vi "Launcher.vi"() -> ()   [LabVIEW 2025]
doc: "This is the top-level VI of this application. When it runs, it behaves like the splash screen many applications use to keep the user occupied while the application loads into memory. This application is quite small, so there is little overhead, which would make the splash screen just flash for a moment. Because that flash is distracting, there is a three-second delay inserted into this VI so that it stays up for a little bit. \n\nThis VI uses a delay-loaded subVI call to load the rest of the application. This trick ensures that the splash screen can load instantly regardless of how large the rest of the VI hierarchy gets, and the loading of the rest of the VIs becomes one step in the load process."
uses:
  Configuration Tools/Config Tool.lvlib
  Configuration Tools/SubVI/Load App.vi
panel:
  out "Engine Status":i32(listbox)=-1
  out "Title":string
  out "String":string
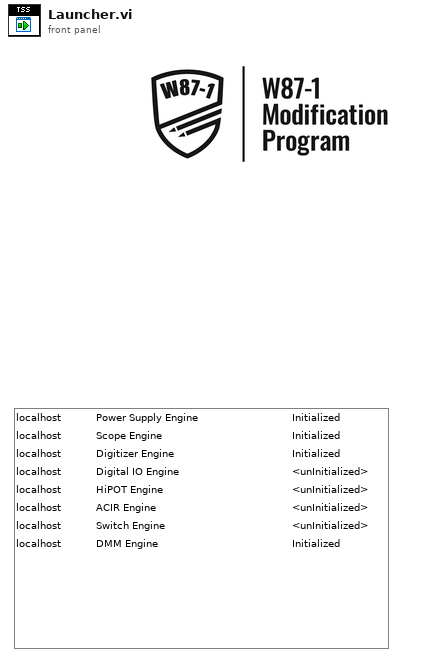
[diagram p1: front panel]
types:
  T1 = enum32{"Invalid", "Default", "Floating", "Floating/Auto-Hide", "Modal"}
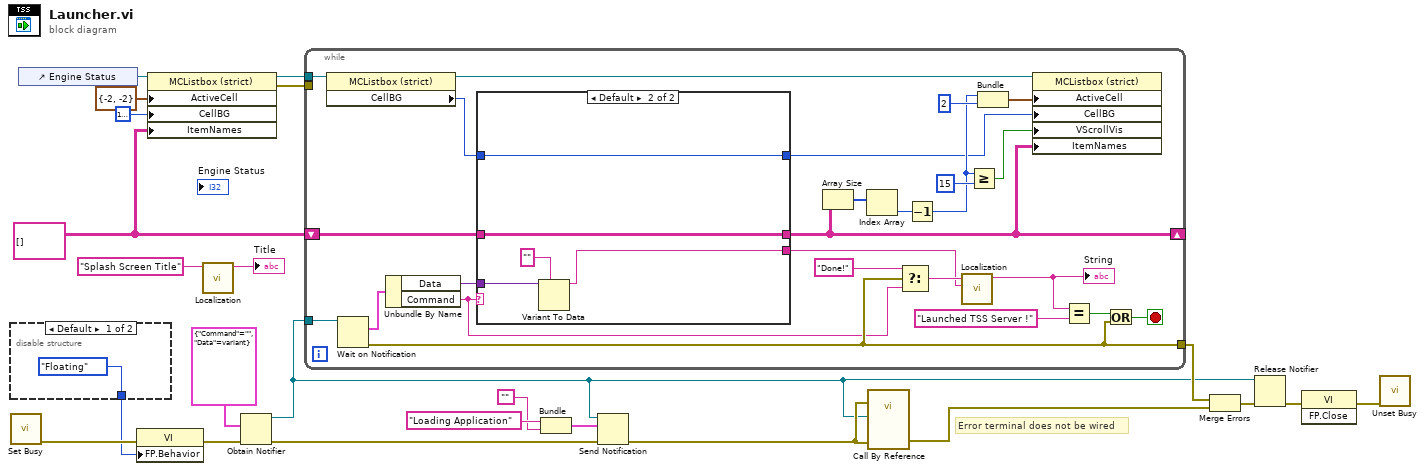
[diagram p0: block diagram]
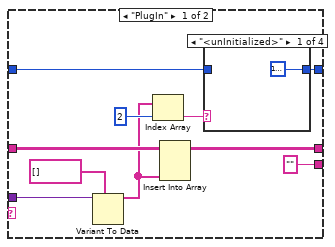
[diagram p2: hidden frame]
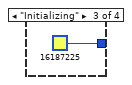
[diagram p4: hidden frame]
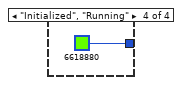
[diagram p5: hidden frame]
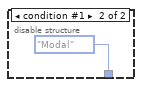
[diagram p6: hidden frame]
diagram:
  w4 = string[][] [] ("ItemNames")
  # "Error terminal does not be wired"
  n1 = disable-structure shown="Default" {
    disable-tunnel: [T1."Floating" ("Front Panel Window:Behavior") T1."Modal" ("Front Panel Window:Behavior")] -> w5
    frame condition #0 (active) {
    }
    frame condition #1 {
    }
  }
  n2 = call <vilib>:"Set Busy.vi"() -> ("error out"=w7:errorcluster)  [unwired: 10 in, 1 out]
  n3 = control-ref of="Engine Status"() -> (w11:refnum<vi>)
  n4 = property class="VI"(error in=w7, "FP.Behavior"=w5) -> (error out=w6:errorcluster)  [unwired: 1 in, 1 out]
  n5 = property class="MCListbox (strict)"(reference=w11, "ActiveCell"=cluster{"Row":i32, "Column":i32} {"Row"=-2, "Column"=-2} ("Active Cell:Active Cell"), "CellBG"=u32 16777216, "ItemNames"=w4) -> (reference out=w10:refnum<vi>, error out=w2:errorcluster)  [unwired: 1 in]
  n6 = call "Localization.vi"("Unlocalized"="Splash Screen Title" ("Window Title")) -> ("Localized"=→"Title":string)  [unwired: 10 in]
  n7 = Obtain Notifier(notification data type=cluster{"Command":string, "Data":variant} {"Command"="", "Data"=variant} ("Message Data"), error in (no error)=w6) -> (notifier out=w3:refnum<notifier>, error out=w16:errorcluster)  [unwired: 2 in, 1 out]
  n8 = while {
    tunnel: w3 -> [w50]
    tunnel: [w27] -> w21
    shift-right: [w34] -> _
    shift-left: w4 -> [w41]
    tunnel: w10 -> [w42]
    tunnel: w2 -> [_]
    stop <- w46 stop-if-true
    n9 = property class="MCListbox (strict)"(reference=w42) -> (reference out=w31:refnum<vi>, "CellBG"=w30:u32)  [unwired: 1 in, 1 out]
    n10 = Wait on Notification(notifier=w50) -> (notification=w43:cluster{"Command":string, "Data":variant}, error out=w27:errorcluster)  [unwired: 3 in, 2 out]
    n11 = Unbundle By Name(w43) -> ("Data"=w29:variant, "Command"=w26:string)
    n12 = case shown="Default" w26 {
      tunnel: w29 -> [w53 w67]
      tunnel: w41 -> [w60 w69]
      tunnel: [w56 w69] -> w34
      tunnel: [w57 w68] -> w32
      tunnel: w30 -> [w55 w68]
      tunnel: ["" ("Type") w65] -> w28
      frame "PlugIn" {
        n13 = Variant To Data(type=string[] [] ("ItemNames"), Variant=w53) -> (data=w52:string[])  [unwired: 1 in, 1 out]
        n14 = Index Array(array=w52, index=2) -> (element=w58:string)
        n15 = Insert Into Array(array=w60, new element=w52) -> (w56:string[][])  [unwired: 2 in]
        n16 = case shown="\"<unInitialized>\"" w58 {
          tunnel: [u32 16777216 w62 u32 16187225 u32 6618880] -> w57
          tunnel: w55 -> [_ w62 _ _]
          frame "<unInitialized>" {
          }
          frame Default {
          }
          frame "Initializing" {
          }
          frame "Initialized", "Running" {
          }
        }
      }
      frame Default {
        n17 = Variant To Data(type="" ("Type"), Variant=w67) -> (data=w65:string)  [unwired: 1 in, 1 out]
      }
    }
    n18 = Array Size(array=w34) -> (size(s)=w37:i32[])
    n19 = Index Array(array=w37) -> (element=w38:i32)  [unwired: 1 in]
    n20 = Select(t="Done!" ("notification"), s=w27, f=w26) -> (s? t:f=w45:string)
    n21 = Decrement(x=w38) -> (x-1=w35:i32)
    n22 = call "Localization.vi"("parameter"=w28, "Unlocalized"=w45) -> ("Localized"=w44:string)  [unwired: 9 in]
    "String" <- w44
    n23 = Greater Or Equal?(x=w35, y=15) -> (x >= y?=w33:bool)
    n24 = Bundle(w35, "disabled index (col)"=2) -> (w40:cluster{i32, "disabled index (col)":i32})  [unwired: 1 in]
    n25 = property class="MCListbox (strict)"(reference=w31, "ActiveCell"=w40, "CellBG"=w32, "VScrollVis"=w33, "ItemNames"=w34) -> ()  [unwired: 1 in, 2 out]
    n26 = Equal?(x=w44, y="Launched TSS Server !" ("notification")) -> (x = y?=w47:bool)
    n27 = Or(x=w47, y=w27) -> (x .or. y?=w46:bool)
  }
  n28 = Bundle("notification"="Loading Application", "") -> (w12:cluster{"notification":string, string})  [unwired: 1 in]
  n29 = Send Notification(notification=w12, notifier=w3, error in (no error)=w16) -> (error out=w19:errorcluster)  [unwired: 1 out]
  n30 = call-by-ref "?"(error in=w19, 8:"error in (no error)"=w19, "notifier"=w3) -> ("error out"=w18:errorcluster)  [unwired: 10 in, 2 out]
  n31 = Merge Errors(w21, w18) -> (w20:errorcluster)
  n32 = Release Notifier(notifier=w3, error in (no error)=w20) -> (error out=w23:errorcluster)  [unwired: 1 in, 2 out]
  n33 = invoke class="VI" method="FP.Close"(error in=w23) -> (error out=w22:errorcluster)  [unwired: 2 in, 2 out]
  n34 = call <vilib>:"Unset Busy.vi"("error in (no error)"=w22) -> ()  [unwired: 10 in, 1 out]
